vi "ErrorHandling.GetErrorHandler.vi"(8 "ErrorIn":errorcluster) -> (0 "ErrorOut":errorcluster, 2 "Found?":bool, 3 "ErrorRef":refnum<data-value>)   [LabVIEW 2016, in "ErrorHandling.lvclass"]
uses:
  ErrorHandling.lvclass
  Package ResourceControl/ObjectHandler/ObjectHandler.GetObjectWType.ctl
  Package ResourceControl/ObjectHandler/ObjectHandler.lvclass
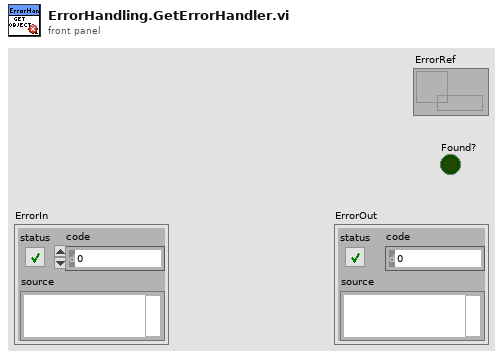
[diagram p1: front panel]
types:
  T1 = typedef "ObjectHandler.lvclass/ObjectHandler.GetObjectWType.ctl" = cluster{"Name":string, "Caller":string}
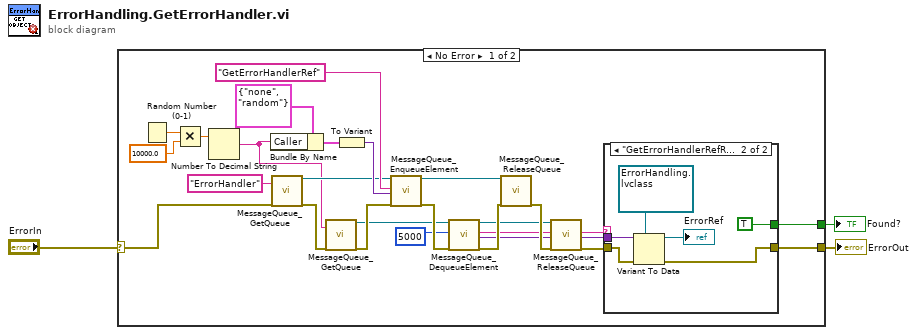
[diagram p0: block diagram]
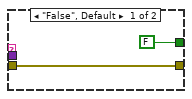
[diagram p2: hidden frame]
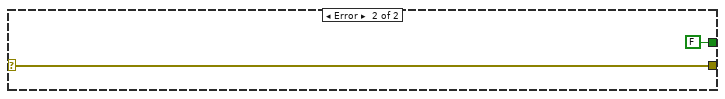
[diagram p3: hidden frame]
diagram:
  n1 = case shown="No Error" "ErrorIn" {
    selector: "ErrorIn" -> [w12 w38]
    tunnel: [w11 w38] -> w3
    tunnel: [w10 FALSE] -> w1
    frame No Error {
      n2 = Random Number (0-1)() -> (number: 0 to 1=w7:dbl)
      n3 = Multiply(x=w7, y=10000.0) -> (x*y=w5:dbl)
      n4 = Number To Decimal String(number=w5) -> (decimal integer string=w4:string)  [unwired: 1 in]
      n5 = Bundle By Name(cluster=T1 {"Name"="none", "Caller"="random"} ("GetRefInput"), "Caller"=w4) -> (w8:T1)
      n6 = call "MessageQueue_GetQueue.vi"("Name"="ErrorHandler", "ErrorIn"=w12) -> ("QueueOut"=w14:refnum<queue>, "ErrorOut"=w15:errorcluster)  [unwired: 15 in, 1 out]
      n7 = call "MessageQueue_GetQueue.vi"("Name"=w4, "ErrorIn"=w15) -> ("QueueOut"=w20:refnum<queue>, "ErrorOut"=w23:errorcluster)  [unwired: 15 in, 1 out]
      n8 = To Variant(anything=w8) -> (Variant=w24:variant)
      n9 = call "MessageQueue_EnqueueElement.vi"("QueueIn"=w14, "Message"="GetErrorHandlerRef", "Data"=w24, "ErrorIn"=w23) -> ("QueueOut"=w17:refnum<queue>, "ErrorOut"=w22:errorcluster)  [unwired: 14 in]
      n10 = call "MessageQueue_DequeueElement.vi"("QueueIn"=w20, "Timeout"=5000, "ErrorIn"=w22) -> ("QueueOut"=w16:refnum<queue>, "Message"=w19:string, "Data"=w18:variant, "ErrorOut"=w28:errorcluster)  [unwired: 12 in, 1 out]
      n11 = call "MessageQueue_ReleaseQueue.vi"("QueueIn"=w17, "ErrorIn"=w28) -> ("ErrorOut"=w27:errorcluster)  [unwired: 15 in, 2 out]
      n12 = call "MessageQueue_ReleaseQueue.vi"("QueueIn"=w16, "ErrorIn"=w27) -> ("ErrorOut"=w13:errorcluster)  [unwired: 15 in, 2 out]
      n13 = case shown="\"GetErrorHandlerRefReturn\"" w19 {
        tunnel: w18 -> [_ w36]
        tunnel: [w29 w31] -> w11
        tunnel: w13 -> [w29 w35]
        tunnel: [FALSE TRUE] -> w10
        frame "False", Default {
        }
        frame "GetErrorHandlerRefReturn" {
          n14 = Variant To Data(error in=w35, type=refnum<data-value> refnum ("data value reference"), Variant=w36) -> (data=→"ErrorRef":refnum<data-value>, error out=w31:errorcluster)
        }
      }
    }
    frame Error {
    }
  }
  "ErrorOut" <- w3
  "Found?" <- w1
